vi "flattenFrequencyToXML.vi"   [LabVIEW 2012, in "UnitsAndXML.lvlib"]
doc: "Generates an XML string for <B>frequency</B> in the unit specified in <B>frequencyUnitInXML</B>. Connect <B>frequency</B> and <B>frequencyAgain</B> to the same source. The VI uses <B>frequencyAgain</B> to obtain the data name."
uses:
  <userlib>/Common/UnitsAndXML/UnitsAndXML.lvlib
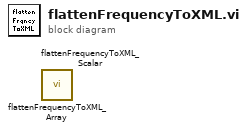
[diagram p0: block diagram]
diagram:
  n1 = call <userlib>:"flattenFrequencyToXML_Array.vi"() -> ()  [unwired: 10 in, 2 out]
  n2 = call <userlib>:"flattenFrequencyToXML_Scalar.vi"() -> ()  [unwired: 10 in, 2 out]
